vi "HFRR ADV v06.vi"() -> ()   [LabVIEW 2025] (continued)
                n1256 = property on="ENTER THE NEW PASSWORD" class="Str"("Visible"=FALSE) -> ()  [unwired: 2 in, 2 out]
              }
              frame True {
                # "password"
                # "change password logic"
                n1257 = local read "ENTER CURRENT PASSWORD"() -> (w2424:string)
                n1258 = local read "dipl pwd"() -> (w2418:string)
                n1259 = String To Byte Array(string=w2424) -> (unsigned byte array=w2426:u8[])
                n1260 = String To Byte Array(string=w2418) -> (unsigned byte array=w2419:u8[])
                n1261 = Array Size(array=w2426) -> (size(s)=w2423:i32)
                n1262 = Array Size(array=w2419) -> (size(s)=w2421:i32)
                n1263 = for {
                  N: w2423 -> [_]
                  tunnel: w2426 -> [w2450]
                  tunnel: [w2448] -> w2427 mode=indexing
                  tunnel: w2423 -> [w2442]
                  i -> [w2443]
                  n1264 = Decrement(x=w2442) -> (x-1=w2440:i32)
                  n1265 = Equal?(x=w2443, y=w2440) -> (x = y?=w2441:bool)
                  n1266 = Index Array(array=w2450, index=w2443) -> (element=w2444:u8)
                  n1267 = Number To Decimal String(number=w2444) -> (decimal integer string=w2449:string)  [unwired: 1 in]
                  n1268 = Select(t="", s=w2441, f="\r") -> (s? t:f=w2446:string)
                  n1269 = Concatenate Strings(w2449, w2446) -> (w2448:string)
                }
                n1270 = for {
                  N: w2421 -> [_]
                  tunnel: w2419 -> [w2438]
                  tunnel: [w2436] -> w2420 mode=indexing
                  tunnel: w2421 -> [w2433]
                  i -> [w2434]
                  n1271 = Decrement(x=w2433) -> (x-1=w2432:i32)
                  n1272 = Equal?(x=w2434, y=w2432) -> (x = y?=w2431:bool)
                  n1273 = Index Array(array=w2438, index=w2434) -> (element=w2437:u8)
                  n1274 = Number To Decimal String(number=w2437) -> (decimal integer string=w2435:string)  [unwired: 1 in]
                  n1275 = Select(t="", s=w2431, f="\r") -> (s? t:f=w2428:string)
                  n1276 = Concatenate Strings(w2435, w2428) -> (w2436:string)
                }
                n1277 = local read "string"() -> (w2425:string)
                n1278 = Concatenate Strings(w2420) -> (w2414:string)
                n1279 = Concatenate Strings(w2425) -> (w2422:string)
                n1280 = Concatenate Strings(w2427) -> (w2415:string)
                n1281 = Equal?(x=w2415, y=w2422) -> (x = y?=w2417:bool)
                n1282 = Equal?(x=w2415, y=w2414) -> (x = y?=w2413:bool)
                n1283 = Or(x=w2417, y=w2413) -> (x .or. y?=w2416:bool)
                n1284 = case shown="True" w2416 {
                  frame False {
                  }
                  frame True {
                    n1285 = property on="ENTER THE NEW PASSWORD" class="Str"("Visible"=TRUE) -> ()  [unwired: 2 in, 2 out]
                  }
                }
              }
            }
          }
          frame #2 {
            n1286 = String To Byte Array(string="ENTER THE NEW PASSWORD") -> (unsigned byte array=w2453:u8[])
            n1287 = Search 1D Array(1D array=w2453, element=u8 10) -> (index of element=w2457:i32)  [unwired: 1 in]
            n1288 = Index Array(array=w2453, index=w2457) -> (element=w2455:u8)
            n1289 = Equal?(x=w2455, y=10) -> (x = y?=w2452:bool)
            n1290 = case shown="False" w2452 {
              frame False {
              }
              frame True {
                n1291 = local write "EDIT"(FALSE) -> ()
                n1292 = local write "SrvM CP"(FALSE) -> ()
                n1293 = local read "ENTER THE NEW PASSWORD"() -> (w2460:string)
                n1294 = String To Byte Array(string=w2460) -> (unsigned byte array=w2465:u8[])
                n1295 = Array Size(array=w2465) -> (size(s)=w2462:i32)
                n1296 = for {
                  N: w2462 -> [_]
                  tunnel: w2465 -> [w2478]
                  tunnel: [w2475] -> w2467 mode=indexing
                  tunnel: w2462 -> [w2470]
                  i -> [w2468]
                  n1297 = Decrement(x=w2470) -> (x-1=w2471:i32)
                  n1298 = Equal?(x=w2468, y=w2471) -> (x = y?=w2472:bool)
                  n1299 = Index Array(array=w2478, index=w2468) -> (element=w2477:u8)
                  n1300 = Number To Decimal String(number=w2477) -> (decimal integer string=w2476:string)  [unwired: 1 in]
                  n1301 = Select(t="", s=w2472, f="\r") -> (s? t:f=w2469:string)
                  n1302 = Concatenate Strings(w2476, w2469) -> (w2475:string)
                }
                n1303 = local read "file path"() -> (w2459:path)
                n1304 = Concatenate Strings(w2467) -> (w2461:string)
                n1305 = Delete(path (use dialog)=w2459) -> (deleted path=w2463:path)  [unwired: 4 in, 2 out]
                n1306 = call <vilib>:"Write Characters To File.vi"("append to file? (new file:F)"=FALSE, "character string"=w2461, "file path (dialog if empty)"=w2463) -> ()  [unwired: 2 in, 1 out]
              }
            }
          }
          frame #3 {
            n1307 = case shown="True" "SrvM CP" {
              frame False {
                w2481 = ""
                n1308 = local write "ENTER CURRENT PASSWORD"(w2481) -> ()
                n1309 = local write "ENTER THE NEW PASSWORD"(w2481) -> ()
                n1310 = property on="ENTER CURRENT PASSWORD" class="Str"("Visible"=FALSE) -> ()  [unwired: 2 in, 2 out]
              }
              frame True {
                n1311 = property on="ENTER THE NEW PASSWORD" class="Str"() -> ("Visible"=w2482:bool)  [unwired: 2 in, 2 out]
                n1312 = Not(x=w2482) -> (.not. x?=w2483:bool)
                n1313 = property on="ENTER CURRENT PASSWORD" class="Str"("Visible"=w2483) -> ()  [unwired: 2 in, 2 out]
              }
            }
          }
          frame #4 {
            n1314 = String To Byte Array(string="Password") -> (unsigned byte array=w2490:u8[])
            n1315 = Search 1D Array(1D array=w2490, element=u8 10) -> (index of element=w2488:i32)  [unwired: 1 in]
            n1316 = Index Array(array=w2490, index=w2488) -> (element=w2489:u8)
            n1317 = Equal?(x=w2489, y=10) -> (x = y?=w2485:bool)
            n1318 = case shown="True" w2485 {
              frame False {
              }
              frame True {
                # "password"
                # "password"
                n1319 = local read "Password"() -> (w2503:string)
                n1320 = String To Byte Array(string=w2503) -> (unsigned byte array=w2506:u8[])
                n1321 = String To Byte Array(string="@143$\n") -> (unsigned byte array=w2492:u8[])
                n1322 = Array Size(array=w2506) -> (size(s)=w2501:i32)
                n1323 = Array Size(array=w2492) -> (size(s)=w2497:i32)
                n1324 = for {
                  N: w2501 -> [_]
                  tunnel: w2506 -> [w2523]
                  tunnel: [w2521] -> w2507 mode=indexing
                  tunnel: w2501 -> [w2518]
                  i -> [w2519]
                  n1325 = Decrement(x=w2518) -> (x-1=w2517:i32)
                  n1326 = Index Array(array=w2523, index=w2519) -> (element=w2522:u8)
                  n1327 = Equal?(x=w2519, y=w2517) -> (x = y?=w2516:bool)
                  n1328 = Number To Decimal String(number=w2522) -> (decimal integer string=w2520:string)  [unwired: 1 in]
                  n1329 = Select(t="", s=w2516, f="\r") -> (s? t:f=w2513:string)
                  n1330 = Concatenate Strings(w2520, w2513) -> (w2521:string)
                }
                n1331 = for {
                  N: w2497 -> [_]
                  tunnel: w2492 -> [w2534]
                  tunnel: [w2532] -> w2495 mode=indexing
                  tunnel: w2497 -> [w2529]
                  i -> [w2530]
                  n1332 = Decrement(x=w2529) -> (x-1=w2528:i32)
                  n1333 = Index Array(array=w2534, index=w2530) -> (element=w2533:u8)
                  n1334 = Equal?(x=w2530, y=w2528) -> (x = y?=w2527:bool)
                  n1335 = Number To Decimal String(number=w2533) -> (decimal integer string=w2531:string)  [unwired: 1 in]
                  n1336 = Select(t="", s=w2527, f="\r") -> (s? t:f=w2524:string)
                  n1337 = Concatenate Strings(w2531, w2524) -> (w2532:string)
                }
                n1338 = local read "file path"() -> (w2491:path)
                n1339 = call <vilib>:"Read Characters From File.vi"("file path (dialog if empty)"=w2491) -> ("character string"=w2505:string)  [unwired: 5 in, 3 out]
                "string" <- w2505
                n1340 = flat-sequence {
                  tunnel: [w2508] -> w2502
                  frame #0 {
                    w2508 = ""
                    n1341 = local write "Password"(w2508) -> ()
                  }
                }
                n1342 = Concatenate Strings(w2495) -> (w2496:string)
                n1343 = Concatenate Strings(w2505) -> (w2504:string)
                n1344 = Concatenate Strings(w2507) -> (w2499:string)
                n1345 = Equal?(x=w2499, y=w2504) -> (x = y?=w2494:bool)
                n1346 = Equal?(x=w2499, y=w2496) -> (x = y?=w2500:bool)
                n1347 = Or(x=w2494, y=w2500) -> (x .or. y?=w2493:bool)
                "x = y?" <- w2493
                n1348 = case shown="False" w2493 {
                  selector: w2493 -> [w2510 _]
                  tunnel: w2502 -> [_ _]
                  frame False {
                    n1349 = And(x=w2510, y=TRUE ("Visible")) -> (x .and. y?=w2511:bool)
                    n1350 = property on="message" class="Str"("Visible"=w2511) -> ()  [unwired: 2 in, 2 out]
                  }
                  frame True {
                    n1351 = property on="message" class="Str"("Visible"=FALSE) -> ()  [unwired: 2 in, 2 out]
                  }
                }
              }
            }
          }
        }
        n1352 = local read "x = y?"() -> (w2350:bool)
        n1353 = local read "HUMIDITY: 2"() -> (w2352:dbl)
        n1354 = local read "HUMIDITY:"() -> (w2351:dbl)
        n1355 = property on="Port 2 Error" class="Clust (strict)"("Visible"="EDIT") -> ()  [unwired: 2 in, 2 out]
        n1356 = property on="Port 1 Error" class="Clust (strict)"("Visible"="EDIT") -> ()  [unwired: 2 in, 2 out]
        n1357 = case shown="True" "SrvM CP 2" {
          frame False {
          }
          frame True {
            n1358 = local write "SrvM CP 2"(FALSE ("SrvM CP 2")) -> ()
            n1359 = local read "HUMIDITY: 2"() -> (w2391:dbl)
            n1360 = local read "TEMP INTERCEPT: 2"() -> (w2390:dbl)
            n1361 = local read "DISPLACEMENT : 4"() -> (w2394:dbl)
            n1362 = local read "TEMPERATURE : 2"() -> (w2393:dbl)
            n1363 = local read "STROKE GAIN : 2"() -> (w2395:dbl)
            n1364 = local read "FRIC. FORCE : 2"() -> (w2396:dbl)
            n1365 = local read "AIR TEMP INTERCEPT: 2"() -> (w2389:dbl)
            n1366 = local read "AIR TEMPERATURE : 2"() -> (w2392:dbl)
            n1367 = local write "HUMIDITY:"(w2391) -> ()
            n1368 = local write "AIR TEMP INTERCEPT:"(w2390) -> ()
            n1369 = local write "TEMPERATURE :"(w2393) -> ()
            n1370 = local write "FRIC. FORCE :"(w2396) -> ()
            n1371 = local write "STROKE GAIN :"(w2395) -> ()
            n1372 = local write "DISPLACEMENT :"(w2394) -> ()
            n1373 = local write "AIR TEMPERATURE :"(w2392) -> ()
            n1374 = local write "TEMP INTERCEPT:"(w2389) -> ()
          }
        }
        n1375 = case shown="True" "SAVE" {
          frame False {
          }
          frame True {
            n1376 = stacked-sequence {
              seq-local: [w2551 _ _] -> [_ w2715 _]
              frame #0 {
                (unwired) i16 5 ("precision (6)")
                # "[CH1]    - FF\n[CH2]   - TEMPERATURE\n[CH3]    - Humidity\n[CH4]    - AIR TEMP\n[CH5]\\- Visa Uno\n[CH6] \\- Visa Due\n[CH7]  \\- file path\n[CH8]   - Displacement Gain\n[CHA]   - Stroke Gain\n[CHB]   - Stroke PID Gain\n[CHC]   -Language Selection\n[CHD]   -Power +\n[CHE]   -Power_\n[CHF]   -Heater\n[CHG]   -Humidity Wet\n[CHH]   -Humidity Dry\n[CHI]   -Integral Time"
                n1377 = local read "Stroke PID Gains"() -> (w2602:T8)
                n1378 = Unbundle By Name(w2602) -> ("Proportional Gain (Kc)"=w2601:dbl, "Integral Time (Ti, min)"=w2543:dbl)
                n1379 = Number To Fractional String(number=w2543, width (-)=i16 10 ("precision (6)"), precision (6)=i16 5) -> (F-format string=w2547:string)  [unwired: 1 in]
                n1380 = local read "Language Selection"() -> (w2599:enum16{"English", "Russian"})
                n1381 = local read "CH-HUMIDITY WET"() -> (w2557:u16)
                n1382 = local read "CH-HUMIDITY DRY"() -> (w2554:u16)
                n1383 = local read "STROKE GAIN :"() -> (w2535:dbl)
                n1384 = local read "CH-POWER +"() -> (w2566:u16)
                n1385 = local read "CH-POWER -"() -> (w2563:u16)
                n1386 = local read "CH-HEATER"() -> (w2560:u16)
                n1387 = local read "AIR TEMPERATURE :"() -> (w2538:dbl)
                n1388 = Concatenate Strings("[CHI]" ("string"), w2547, "-Integral Time " ("string"), "\r") -> (w2544:string)
                n1389 = local read "DISPLACEMENT :"() -> (w2536:dbl)
                n1390 = local read "TEMPERATURE :"() -> (w2539:dbl)
                n1391 = local read "FRIC. FORCE :"() -> (w2540:dbl)
                n1392 = local read "HUMIDITY:"() -> (w2537:dbl)
                n1393 = Path To String(path="File Path") -> (string=w2624:string)
                n1394 = Number To Fractional String(number=w2535, width (-)=i16 10 ("precision (6)"), precision (6)=i16 5) -> (F-format string=w2615:string)  [unwired: 1 in]
                n1395 = Number To Fractional String(number=w2601, width (-)=i16 10 ("precision (6)"), precision (6)=i16 5) -> (F-format string=w2603:string)  [unwired: 1 in]
                n1396 = Number To Fractional String(number=w2599, width (-)=i16 10 ("precision (6)"), precision (6)=i16 5) -> (F-format string=w2595:string)  [unwired: 1 in]
                n1397 = Number To Fractional String(number=w2566, width (-)=i16 10 ("precision (6)"), precision (6)=i16 5) -> (F-format string=w2589:string)  [unwired: 1 in]
                n1398 = Number To Fractional String(number=w2563, width (-)=i16 10 ("precision (6)"), precision (6)=i16 5) -> (F-format string=w2586:string)  [unwired: 1 in]
                n1399 = Number To Fractional String(number=w2560, width (-)=i16 10 ("precision (6)"), precision (6)=i16 5) -> (F-format string=w2581:string)  [unwired: 1 in]
                n1400 = Number To Fractional String(number=w2557, width (-)=i16 10 ("precision (6)"), precision (6)=i16 5) -> (F-format string=w2578:string)  [unwired: 1 in]
                n1401 = Number To Fractional String(number=w2554, width (-)=i16 10 ("precision (6)"), precision (6)=i16 5) -> (F-format string=w2573:string)  [unwired: 1 in]
                n1402 = local read "Com Port 1"() -> (w2542:refnum<visa-resource-name>)
                n1403 = local read "Com Port 2"() -> (w2541:refnum<visa-resource-name>)
                n1404 = Concatenate Strings(w2624, "\\" ("string")) -> (w2623:string)
                n1405 = Number To Fractional String(number=w2540, width (-)=i16 10 ("precision (6)"), precision (6)=i16 5) -> (F-format string=w2656:string)  [unwired: 1 in]
                n1406 = Number To Fractional String(number=w2539, width (-)=i16 10 ("precision (6)"), precision (6)=i16 5) -> (F-format string=w2655:string)  [unwired: 1 in]
                n1407 = Number To Fractional String(number=w2537, width (-)=i16 10 ("precision (6)"), precision (6)=i16 5) -> (F-format string=w2649:string)  [unwired: 1 in]
                n1408 = Number To Fractional String(number=w2538, width (-)=i16 10 ("precision (6)"), precision (6)=i16 5) -> (F-format string=w2643:string)  [unwired: 1 in]
                n1409 = Number To Fractional String(number=w2536, width (-)=i16 10 ("precision (6)"), precision (6)=i16 5) -> (F-format string=w2616:string)  [unwired: 1 in]
                n1410 = Concatenate Strings("[CHA]" ("string"), w2615, "- Stroke Gain" ("string"), "\r") -> (w2609:string)
                n1411 = Concatenate Strings("[CHB]" ("string"), w2603, "- Stroke PID Gain" ("string"), "\r") -> (w2600:string)
                n1412 = Concatenate Strings("[CHC]" ("string"), w2595, "-Language Selection" ("string"), "\r") -> (w2592:string)
                n1413 = Concatenate Strings("[CHD]" ("string"), w2589, "-Power +" ("string"), "\r") -> (w2571:string)
                n1414 = Concatenate Strings("[CHG]" ("string"), w2578, "-Humidity Wet" ("string"), "\r") -> (w2568:string)
                n1415 = Concatenate Strings("[CHH]" ("string"), w2573, "-Humidity Dry" ("string"), "\r") -> (w2567:string)
                n1416 = Concatenate Strings("[CH1]" ("string"), w2656, " - FF" ("string"), "\r") -> (w2654:string)
                n1417 = Concatenate Strings("[CH2]" ("string"), w2655, " - TEMPERATURE" ("string"), "\r") -> (w2653:string)
                n1418 = Concatenate Strings("[CH3]" ("string"), w2649, " - Humidity" ("string"), "\r") -> (w2646:string)
                n1419 = Concatenate Strings("[CH4]" ("string"), w2643, " - AIR TEMP" ("string"), "\r") -> (w2639:string)
                n1420 = Concatenate Strings("[CH5]" ("string"), w2542, "- Visa Uno" ("string"), "\r") -> (w2632:string)
                n1421 = Concatenate Strings("[CH6]" ("string"), w2541, "- Visa Due" ("string"), "\r") -> (w2627:string)
                n1422 = Concatenate Strings("[CH7]" ("string"), w2623, "- file path" ("string"), "\r") -> (w2626:string)
                n1423 = Concatenate Strings("[CH8]" ("string"), w2616, "- Displacement Gain" ("string"), "\r") -> (w2619:string)
                n1424 = Concatenate Strings("[CHE]" ("string"), w2586, "-Power_" ("string"), "\r") -> (w2570:string)
                n1425 = Concatenate Strings("[CHF]" ("string"), w2581, "-Heater" ("string"), "\r") -> (w2569:string)
                n1426 = Concatenate Strings(w2654, w2653, w2646, w2639, w2632, w2627, w2626, w2619, w2609, w2600, w2592, w2571, w2570, w2569, w2568, w2567, w2544) -> (w2551:string)
                "gain" <- w2551
              }
              frame #1 {
                n1427 = local read "Camera Port :"() -> (w2668:string)
                n1428 = local read "TEMP INTERCEPT:"() -> (w2677:dbl)
                n1429 = local read "Humidity :"() -> (w2676:refnum<visa-resource-name>)
                n1430 = local read "AIR TEMP INTERCEPT:"() -> (w2678:dbl)
                n1431 = local read "LvdtOff"() -> (w2680:dbl)
                n1432 = Number To Fractional String(number=w2677, width (-)=i16 10 ("precision (6)"), precision (6)=i16 5) -> (F-format string=w2703:string)  [unwired: 1 in]
                n1433 = local read "Com Port 3"() -> (w2687:refnum<visa-resource-name>)
                n1434 = Concatenate Strings("[CH8]" ("string"), w2668, "- Visa Camera" ("string"), "\r") -> (w2667:string)
                n1435 = Concatenate Strings("[CH7]" ("string"), w2676, "- Visa Humidity" ("string"), "\r") -> (w2672:string)
                n1436 = Number To Fractional String(number=w2678, width (-)=i16 10 ("precision (6)"), precision (6)=i16 5) -> (F-format string=w2710:string)  [unwired: 1 in]
                n1437 = Number To Fractional String(number=w2680, width (-)=i16 10 ("precision (6)"), precision (6)=i16 5) -> (F-format string=w2684:string)  [unwired: 1 in]
                n1438 = Concatenate Strings("[CHK]" ("string"), w2703, "-TEMP INTERCEPT" ("string"), "\r") -> (w2699:string)
                n1439 = Concatenate Strings("[SNO]" ("string"), "S.NO", "-" ("string"), "\r") -> (w2695:string)
                n1440 = Concatenate Strings("[CHI]" ("string"), w2684, "-LVDT Position Offset" ("string"), "\r") -> (w2679:string)
                n1441 = Concatenate Strings("[CHJ]" ("string"), w2710, "-AIR TEMP INTERCEPT" ("string"), "\r") -> (w2700:string)
                n1442 = Concatenate Strings("[CHL]" ("string"), w2687, "- Visa humid" ("string"), "\r") -> (w2690:string)
                n1443 = String To Path(string="C:\\LAB-IQ\\calibrate WO 2464.dcf") -> (path=w2688:path)
                n1444 = Concatenate Strings(w2715, w2700, w2699, w2695, w2690, w2679, w2672, w2667) -> (w2714:string)
                n1445 = call <vilib>:"Write Characters To File.vi"("append to file? (new file:F)"=FALSE, "character string"=w2714, "file path (dialog if empty)"=w2688) -> ()  [unwired: 2 in, 1 out]
              }
              frame #2 {
                n1446 = local write "Lan flag"(0.0 ("Lan flag")) -> ()
                n1447 = local write "conststatus"(0.0 ("rpm value : 2")) -> ()
                n1448 = local write "SAVE"(FALSE ("OK Button 14")) -> ()
                n1449 = local write "Re-Initialise"(TRUE ("Re-Initialise")) -> ()
              }
            }
          }
        }
        n1450 = And(x="EDIT", y=w2350) -> (x .and. y?=w2348:bool)
        n1451 = local read "DISPLACEMENT : 4"() -> (w2361:dbl)
        n1452 = local read "TEMPERATURE : 2"() -> (w2359:dbl)
        n1453 = local read "STROKE GAIN : 2"() -> (w2365:dbl)
        n1454 = local read "DISPLACEMENT :"() -> (w2360:dbl)
        n1455 = local read "FRIC. FORCE : 2"() -> (w2368:dbl)
        n1456 = local read "TEMPERATURE :"() -> (w2357:dbl)
        n1457 = local read "STROKE GAIN :"() -> (w2364:dbl)
        n1458 = local read "FRIC. FORCE :"() -> (w2367:dbl)
        n1459 = case shown="False" w2348 {
          tunnel: [u8 2 ("Disabled") u8 0 ("Disabled")] -> w2347
          tunnel: [w2720 TRUE ("Visible")] -> w2346
          frame False {
            w2720 = FALSE ("Visible")
            n1460 = local write "EDIT 2"(w2720) -> ()
          }
          frame True {
          }
        }
        n1461 = Subtract(x=w2352, y=w2351) -> (x-y=w2353:dbl)
        n1462 = local read "AIR TEMPERATURE : 2"() -> (w2356:dbl)
        n1463 = local read "AIR TEMPERATURE :"() -> (w2355:dbl)
        n1464 = Divide(x=w2353, y=w2351) -> (x/y=w2375:dbl)
        n1465 = Subtract(x=w2368, y=w2367) -> (x-y=w2366:dbl)
        n1466 = Subtract(x=w2359, y=w2357) -> (x-y=w2358:dbl)
        n1467 = Subtract(x=w2365, y=w2364) -> (x-y=w2363:dbl)
        n1468 = Subtract(x=w2361, y=w2360) -> (x-y=w2362:dbl)
        n1469 = Subtract(x=w2356, y=w2355) -> (x-y=w2354:dbl)
        n1470 = Divide(x=w2366, y=w2367) -> (x/y=w2386:dbl)
        n1471 = Divide(x=w2358, y=w2357) -> (x/y=w2379:dbl)
        n1472 = Divide(x=w2363, y=w2364) -> (x/y=w2383:dbl)
        n1473 = Divide(x=w2362, y=w2360) -> (x/y=w2382:dbl)
        n1474 = Multiply(x=w2375, y=100.0) -> (x*y=→"HUMIDITY  Calibration Error":dbl)
        n1475 = Divide(x=w2354, y=w2355) -> (x/y=w2378:dbl)
        n1476 = Multiply(x=w2386, y=100.0) -> (x*y=→"FRIC. FORCE Calibration Error":dbl)
        n1477 = Multiply(x=w2379, y=100.0) -> (x*y=→"TEMPERATURE  Calibration Error":dbl)
        n1478 = Multiply(x=w2383, y=100.0) -> (x*y=→"STROKE Calibration Error":dbl)
        n1479 = Multiply(x=w2382, y=100.0) -> (x*y=→"DISPLACEMENT  Calibration Error":dbl)
        n1480 = property on="EDIT 2" class="Bool (strict)"("Visible"=w2346) -> ()  [unwired: 2 in, 2 out]
        n1481 = property on="SAVE" class="Bool (strict)"("Visible"=w2346) -> ()  [unwired: 2 in, 2 out]
        n1482 = property on="SrvM CP" class="Bool (strict)"("Disabled"=w2347) -> ()  [unwired: 2 in, 2 out]
        n1483 = property on="visa due" class="CmbBox"("Disabled"=w2347) -> ()  [unwired: 2 in, 2 out]
        n1484 = property on="LvdtOff" class="DigNum (strict)"("Disabled"=w2347) -> ()  [unwired: 2 in, 2 out]
        n1485 = property on="File Path" class="Path"("Disabled"=w2347) -> ()  [unwired: 2 in, 2 out]
        n1486 = Multiply(x=w2378, y=100.0) -> (x*y=→"AIR TEMPERATURE  Calibration Error":dbl)
        n1487 = property on="Tab Control" class="TabCtl (strict)"("Visible"=w2346) -> ()  [unwired: 2 in, 2 out]
        n1488 = property on="Language Selection" class="Enum (strict)"("Visible"=w2346) -> ()  [unwired: 2 in, 2 out]
        n1489 = property on="Tab Control 7" class="TabCtl (strict)"("Disabled"=w2347) -> ()  [unwired: 2 in, 2 out]
        n1490 = property on="AIR TEMP INTERCEPT:" class="DigNum (strict)"("Disabled"=w2347) -> ()  [unwired: 2 in, 2 out]
        n1491 = property on="CH-POWER -" class="DigNum (strict)"("Disabled"=w2347) -> ()  [unwired: 2 in, 2 out]
        n1492 = property on="CH-POWER +" class="DigNum (strict)"("Disabled"=w2347) -> ()  [unwired: 2 in, 2 out]
        n1493 = property on="AIR TEMPERATURE :" class="DigNum (strict)"("Disabled"=w2347) -> ()  [unwired: 2 in, 2 out]
        n1494 = property on="STROKE GAIN :" class="DigNum (strict)"("Disabled"=w2347) -> ()  [unwired: 2 in, 2 out]
        n1495 = property on="SPEED OUT:" class="DigNum (strict)"("Disabled"=w2347) -> ()  [unwired: 2 in, 2 out]
        n1496 = property on="CH-HUMIDITY DRY" class="DigNum (strict)"("Disabled"=w2347) -> ()  [unwired: 2 in, 2 out]
        n1497 = property on="HUMIDITY:" class="DigNum (strict)"("Disabled"=w2347) -> ()  [unwired: 2 in, 2 out]
        n1498 = property on="CH-HUMIDITY WET" class="DigNum (strict)"("Disabled"=w2347) -> ()  [unwired: 2 in, 2 out]
        n1499 = property on="Stroke PID Gains" class="Clust (strict)"("Disabled"=w2347) -> ()  [unwired: 2 in, 2 out]
        n1500 = property on="TEMPERATURE :" class="DigNum (strict)"("Disabled"=w2347) -> ()  [unwired: 2 in, 2 out]
        n1501 = property on="DISPLACEMENT :" class="DigNum (strict)"("Disabled"=w2347) -> ()  [unwired: 2 in, 2 out]
        n1502 = property on="CH-HEATER" class="DigNum (strict)"("Disabled"=w2347) -> ()  [unwired: 2 in, 2 out]
        n1503 = property on="TEMP INTERCEPT:" class="DigNum (strict)"("Disabled"=w2347) -> ()  [unwired: 2 in, 2 out]
        n1504 = property on="FRIC. FORCE :" class="DigNum (strict)"("Disabled"=w2347) -> ()  [unwired: 2 in, 2 out]
      }
    }
    n1505 = local read "Re-Initialise"() -> (w1729:bool)
    n1506 = local read "Main Tab"() -> (w1725:T2)
    n1507 = local read "service 3"() -> (w1726:bool)
    n1508 = local read "OPEN 6"() -> (w1728:bool)
    n1509 = local read "EDIT 2"() -> (w1731:bool)
    n1510 = local read "RUN"() -> (w1743:bool)
    n1511 = local read "RUN"() -> (w1741:bool)
    n1512 = disable-structure shown="Disabled" {
      disable-tunnel: [w1758 _] -> w1723
      disable-tunnel: [w1757 _] -> w1721
      frame Disabled {
        n1513 = local read "Temperature before test"() -> (w1751:dbl)
        n1514 = local read "Temperature after test"() -> (w1764:dbl)
        n1515 = case shown="True" "Save Results" {
          frame False {
          }
          frame True {
            w1780 = "\r"
            n1516 = local write "Save Results"(FALSE ("OK Button 5")) -> ()
            n1517 = local read "Temperature before test"() -> (w1818:dbl)
            n1518 = local read "Temperature after test"() -> (w1820:dbl)
            n1519 = local read "Humidity before test"() -> (w1817:dbl)
            n1520 = local read "Humidity after test"() -> (w1819:dbl)
            n1521 = local read "WS1.4"() -> (w1824:dbl)
            n1522 = local read "AVP"() -> (w1822:dbl)
            n1523 = Number To Fractional String(number=w1824, width (-)=i16 6, precision (6)=i16 1) -> (F-format string=w1784:string)  [unwired: 1 in]
            n1524 = local read "MWSD"() -> (w1821:dbl)
            n1525 = local read "String"() -> (w1813:string)
            n1526 = local read "FILE"() -> (w1816:string)
            n1527 = local read "HCF"() -> (w1823:dbl)
            n1528 = Number To Fractional String(number=w1817, width (-)=i16 6, precision (6)=i16 1) -> (F-format string=w1809:string)  [unwired: 1 in]
            n1529 = Number To Fractional String(number=w1818, width (-)=i16 6, precision (6)=i16 1) -> (F-format string=w1806:string)  [unwired: 1 in]
            n1530 = Number To Fractional String(number=w1819, width (-)=i16 6, precision (6)=i16 1) -> (F-format string=w1802:string)  [unwired: 1 in]
            n1531 = Number To Fractional String(number=w1820, width (-)=i16 6, precision (6)=i16 1) -> (F-format string=w1798:string)  [unwired: 1 in]
            n1532 = Number To Fractional String(number=w1822, width (-)=i16 6, precision (6)=i16 3) -> (F-format string=w1791:string)  [unwired: 1 in]
            n1533 = Concatenate Strings(w1813, w1816) -> (w1835:string)
            n1534 = Number To Fractional String(number=w1821, width (-)=i16 6, precision (6)=i16 1) -> (F-format string=w1795:string)  [unwired: 1 in]
            n1535 = Number To Fractional String(number=w1823, width (-)=i16 6, precision (6)=i16 2) -> (F-format string=w1789:string)  [unwired: 1 in]
            n1536 = Concatenate Strings("(" ("string"), w1784, ")Microns" ("string")) -> (w1783:string)
            n1537 = local read "REMARKS"() -> (w1815:string)
            "REMARKS 2" <- w1815
            n1538 = Concatenate Strings("(" ("string"), w1809, " ) % RH," ("string")) -> (w1810:string)
            n1539 = Concatenate Strings(w1789, ")" ("string")) -> (w1787:string)
            n1540 = Concatenate Strings("(" ("string"), w1806, ")  Deg C ," ("string")) -> (w1805:string)
            n1541 = Concatenate Strings("(" ("string"), w1802, " ) % RH," ("string")) -> (w1801:string)
            n1542 = Concatenate Strings("(" ("string"), w1798, ")  Deg C ," ("string")) -> (w1797:string)
            n1543 = Concatenate Strings("(" ("string"), w1795, ")  Microns," ("string")) -> (w1794:string)
            n1544 = Concatenate Strings("(" ("string"), w1791, ")  kPa," ("string")) -> (w1781:string)
            n1545 = Concatenate Strings(w1835, ".dwm" ("Substring")) -> (w1833:string)
            n1546 = String To Path(string=w1833) -> (path=w1832:path)
            n1547 = Concatenate Strings(w1815, w1780, " Humidity before test= " ("Substring"), w1810, w1780, " Temperature before test = " ("Substring"), w1805, w1780, " Humidity after test= " ("Substring"), w1801, w1780, "Temperature after test = " ("Substring"), w1797, w1780, "MSD = " ("Substring"), w1794, w1780, "  AVP = " ("Substring"), w1781, w1780, "  HCF                     =( " ("Substring"), w1787, w1780, " WS1.4                  = " ("Substring"), w1783, w1780) -> (w1779:string)
            "data" <- w1779
            n1548 = call <vilib>:"Write Characters To File.vi"("append to file? (new file:F)"=FALSE, "character string"=w1779, "file path (dialog if empty)"=w1832) -> ()  [unwired: 2 in, 1 out]
            n1549 = Match Pattern(string=w1779, regular expression="!") -> (after substring=→"export":string)  [unwired: 1 in, 3 out]
          }
        }
        n1550 = Add(x=231.864, y=w1751) -> (x+y=w1748:dbl)
        n1551 = Add(x=231.864, y=w1764) -> (x+y=w1761:dbl)
        n1552 = Divide(x=1705.984, y=w1748) -> (x/y=w1749:dbl)
        n1553 = Divide(x=1705.984, y=w1761) -> (x/y=w1762:dbl)
        n1554 = local read "Humidity before test"() -> (w1753:dbl)
        n1555 = local read "Humidity after test"() -> (w1766:dbl)
        n1556 = Subtract(x=8.017352 ("y"), y=w1749) -> (x-y=w1775:dbl)
        n1557 = Subtract(x=8.017352 ("y"), y=w1762) -> (x-y=w1769:dbl)
        n1558 = expression code="10**y"(w1775) -> (w1755:dbl)
        n1559 = expression code="10**y"(w1769) -> (w1768:dbl)
        n1560 = Multiply(x=w1753, y=w1755) -> (x*y=w1754:dbl)
        n1561 = Multiply(x=w1766, y=w1768) -> (x*y=w1767:dbl)
        n1562 = Divide(x=w1754, y=750.0) -> (x/y=w1770:dbl)
        n1563 = Divide(x=w1767, y=750.0) -> (x/y=w1771:dbl)
        n1564 = Add(x=w1770, y=w1771) -> (x+y=w1772:dbl)
        n1565 = Divide(x=w1772, y=2.0) -> (x/y=w1774:dbl)
        n1566 = local write "AVP"(w1774) -> ()
        n1567 = Subtract(x=1.4, y=w1774) -> (x-y=w1757:dbl)
        n1568 = local read "HCF"() -> (w1758:dbl)
      }
      frame Enabled {
      }
    }
    n1569 = case shown="True" "EDIT 3" {
      frame False {
      }
      frame True {
        n1570 = local write "EDIT 3"(FALSE ("EDIT 3")) -> ()
        n1571 = local write "Main Tab"(T2."About" ("Main Tab")) -> ()
      }
    }
    n1572 = case shown="True" w1729 {
      frame False {
      }
      frame True {
        n1573 = local write "Re-Initialise"(FALSE ("Re-Initialise")) -> ()
      }
    }
    n1574 = case shown="False" w1743 {
      frame False {
        n1575 = local read "stopT"() -> (w2729:bool)
        n1576 = case shown="True" w2729 {
          frame False {
          }
          frame True {
            w2730 = FALSE
            n1577 = local write "stopT"(w2730) -> ()
            n1578 = local write "st enable"(w2730) -> ()
          }
        }
      }
      frame True {
        "stopT" <- TRUE
      }
    }
    n1579 = case shown="True" w1741 {
      frame False {
      }
      frame True {
        n1580 = local read "Main Tab"() -> (w2727:T2)
        n1581 = case shown="\"Compare Files\"" w2727 {
          frame "Acquire", Default {
          }
          frame "Compare Files" {
            n1582 = local write "Main Tab"(T2."Acquire" ("Main Tab")) -> ()
          }
          frame "About" {
          }
        }
      }
    }
    n1583 = case shown="True" w1731 {
      frame False {
        n1584 = property on="Password 2" class="Str"("Visible"=FALSE) -> ()  [unwired: 2 in, 2 out]
        n1585 = local write "Password 2"("" ("Password")) -> ()
      }
      frame True {
        n1586 = property on="Password 2" class="Str"("Visible"=TRUE) -> ()  [unwired: 2 in, 2 out]
        n1587 = Equal?(x="Password 2", y="HFRR1234") -> (x = y?=w1864:bool)
        n1588 = case shown="True" w1864 {
          tunnel: "Password 2" -> [w1867 _]
          frame False {
            n1589 = String Length(string=w1867) -> (length=w1868:i32)
            n1590 = Greater Than 0?(x=w1868) -> (x > 0?=w1866:bool)
            n1591 = case shown="False" w1866 {
              frame False {
                n1592 = property on="Password 2" class="Str"("Caption.Text"="Password (Advance Setting)") -> ()  [unwired: 2 in, 2 out]
              }
              frame True {
                n1593 = property on="Password 2" class="Str"("Caption.Text"="Incorrect Password!") -> ()  [unwired: 2 in, 2 out]
              }
            }
          }
          frame True {
            n1594 = local write "EDIT 2"(FALSE ("EDIT 2")) -> ()
            n1595 = local write "Password 2"("" ("Password")) -> ()
            n1596 = local write "Main Tab"(T2."Advance" ("Main Tab")) -> ()
          }
        }
      }
    }
    n1597 = case shown="True" "Prog Uno" {
      frame False {
      }
      frame True {
        n1598 = stacked-sequence {
          frame #0 {
            n1599 = Delete(path (use dialog)=path "C:/LAB-IQ-NXT/UNOCOMPILE.bat" ("working directory")) -> ()  [unwired: 4 in, 3 out]
          }
          frame #1 {
            n1600 = local read "Com Port 1"() -> (w2328:refnum<visa-resource-name>)
            n1601 = Concatenate Strings("cmd.exe /c \"mode " ("command line"), w2328, ":1200,n,8,1\"\n" ("command line")) -> (w2333:string)
            n1602 = Concatenate Strings(w2333, "CD\\\nCD WinDucom\navrdude -C avrdude.conf -v -patmega328p -carduino -P" ("command line"), w2328, " -b115200 -D -Uflash:w:UNO_V20.hex:i\n" ("command line"), "\r") -> (w2335:string)
            "STR" <- w2335
            n1603 = call <vilib>:"Write Characters To File.vi"("append to file? (new file:F)"=FALSE, "character string"=w2335, "file path (dialog if empty)"=path "C:/LAB-IQ-NXT/UNOCOMPILE.bat" ("working directory")) -> ()  [unwired: 2 in, 1 out]
          }
          frame #2 {
            n1604 = disable-structure shown="Disabled" {
              frame Disabled {
                w2339 = "cmd.exe  /c \"C:\\LAB-IQ-NXT\\UNOCOMPILE.bat\"" ("string")
                n1605 = local write "Prog Uno"(FALSE ("run minimized? (F)")) -> ()
                n1606 = call <vilib>:"System Exec.vi"("expected output size  (4096)"=u32 65535, "run minimized? (F)"=FALSE, "wait until completion? (T)"=TRUE ("run minimized? (F)"), "working directory"=path "C:/LAB-IQ-NXT", "standard input"=w2339, "command line"=w2339) -> ("error out"=w2338:errorcluster, "standard output"=→"String 42":string)  [unwired: 2 in, 2 out]
                "error out 3" <- w2338
                n1607 = flat-sequence {
                  tunnel: w2338 -> [_]
                  frame #0 {
                  }
                }
              }
              frame Enabled {
              }
            }
          }
        }
      }
    }
    n1608 = case shown="\"ASTM D6079\", Default" "TEST STANDARD" {
      tunnel: [2.0 ("Set Temp") 0.0 ("Set Temp") 2.0 ("Set Temp") 0.0 ("Set Temp")] -> w1732
      frame "ASTM D6079", Default {
        w2285 = 50.0 ("Hz")
        w2286 = 53.0 ("Set Rh")
        w2288 = 1.0 ("Set Strk")
        w2287 = 60.0 ("Set Temp")
        # "astm hide"
        n1609 = local write "NORMAL LOAD"(2.0 ("NORMAL LOAD")) -> ()
        n1610 = local write "Set Strk"(w2288) -> ()
        n1611 = local write "Set Hz"(w2285) -> ()
        n1612 = local write "Set Temp"(w2287) -> ()
        n1613 = local write "Set Rh"(w2286) -> ()
        n1614 = local write "test time"(75.0 ("test time")) -> ()
        n1615 = local write "Set Stroke:"(w2288) -> ()
        n1616 = local write "Set Humidity:"(w2286) -> ()
        n1617 = local write "Set Frequency:"(w2285) -> ()
        n1618 = local write "Set Temperature:"(w2287) -> ()
        "Test Standard" <- "ASTM D6079" ("Test Standard 2")
      }
      frame "ISO 12156" {
        n1619 = local write "Set Strk"(1.0 ("Set Strk")) -> ()
        n1620 = local write "NORMAL LOAD"(2.0 ("NORMAL LOAD")) -> ()
        n1621 = local write "Set Temp"(60.0 ("Set Temp")) -> ()
        n1622 = local write "test time"(75.0 ("test time")) -> ()
        n1623 = local write "Set Hz"(50.0 ("Hz")) -> ()
        n1624 = local write "Set Rh"(53.0 ("Set Rh")) -> ()
      }
      frame "CEC F-096-A-06" {
        n1625 = local write "Set Strk"(1.0 ("Set Strk")) -> ()
        n1626 = local write "NORMAL LOAD"(2.0 ("NORMAL LOAD")) -> ()
        n1627 = local write "Set Temp"(60.0 ("Set Temp")) -> ()
        n1628 = local write "test time"(75.0 ("test time")) -> ()
        n1629 = local write "Set Hz"(50.0 ("Hz")) -> ()
        n1630 = local write "Set Rh"(53.0 ("Set Rh")) -> ()
      }
      frame "Custom" {
      }
    }
    n1631 = case shown="True" "Prog Due" {
      frame False {
      }
      frame True {
        n1632 = stacked-sequence {
          frame #0 {
            n1633 = Delete(path (use dialog)=path "C:/LAB-IQ/DUECOMPILE.bat" ("working directory")) -> ()  [unwired: 4 in, 3 out]
          }
          frame #1 {
            n1634 = disable-structure shown="Disabled" {
              frame Disabled {
                n1635 = local read "visa due"() -> (w2310:string)
                n1636 = Concatenate Strings("cmd.exe /c \"mode " ("command line"), w2310, ":1200,n,8,1\"\n" ("command line")) -> (w2315:string)
                n1637 = Concatenate Strings(w2315, "CD\\\nCD WinDucom\nTIMEOUT 1\n bossac.exe -i -d --port=" ("command line"), w2310, " -U false -e -w -v -b DUE.bin -R\n" ("command line"), "\r") -> (w2317:string)
                "concatenated string 2" <- w2317
                n1638 = call <vilib>:"Write Characters To File.vi"("append to file? (new file:F)"=FALSE, "character string"=w2317, "file path (dialog if empty)"=path "C:/LAB-IQ-NXT/DUECOMPILE.bat" ("working directory")) -> ()  [unwired: 2 in, 1 out]
              }
              frame Enabled {
              }
            }
          }
          frame #2 {
            # "C:\\LAB-IQ-NXT\\DUECOMPILE.bat"
            n1639 = disable-structure shown="Disabled" {
              frame Disabled {
                w2322 = "cmd.exe  /c \"C:\\LAB-IQ-NXT\\DUECOMPILE.bat\"" ("string")
                n1640 = call <vilib>:"System Exec.vi"("expected output size  (4096)"=u32 65535, "run minimized? (F)"=FALSE, "wait until completion? (T)"=TRUE ("run minimized? (F)"), "working directory"=path "C:/LAB-IQ-NXT", "standard input"=w2322, "command line"=w2322) -> ("error out"=w2321:errorcluster, "standard output"=→"String 44":string)  [unwired: 2 in, 2 out]
                "error out 4" <- w2321
                n1641 = flat-sequence {
                  tunnel: w2321 -> [_]
                  frame #0 {
                  }
                }
              }
              frame Enabled {
              }
            }
            n1642 = local write "Prog Due"(FALSE ("Prog Due")) -> ()
          }
        }
      }
    }
    n1643 = Or(x=w1728, y=w1726) -> (x .or. y?=w1727:bool)
    n1644 = case shown="\"About\"" w1725 {
      tunnel: [T18."Acquire" ("Main Tab") T18."Compare Files" ("Main Tab") T18."About" ("Main Tab")] -> w1739
      frame "Acquire", Default {
      }
      frame "Compare Files" {
      }
      frame "About" {
      }
    }
    n1645 = Or(x=w1733, y="OPEN") -> (x .or. y?=w1734:bool)
    n1646 = case shown="True" w1734 {
      tunnel: w1733 -> [_ w1874]
      frame False {
      }
      frame True {
        n1647 = stacked-sequence {
          tunnel: w1874 -> [_ w1941 _ _]
          frame #0 {
            w1890 = "  " ("String 6")
            n1648 = local write "OPEN"(FALSE ("open")) -> ()
            n1649 = local read "string1 2"() -> (w1878:string)
            n1650 = local read "string1 3"() -> (w1877:string)
            n1651 = local read "string1 4"() -> (w1876:string)
            n1652 = property on="OPEN" class="Bool (strict)"("Visible"=FALSE) -> ()  [unwired: 2 in, 2 out]
            n1653 = local write "String 6"(w1890) -> ()
            n1654 = local write "String 7"(w1890) -> ()
            n1655 = local write "String 8"(w1890) -> ()
            n1656 = local write "String 12"(w1890) -> ()
            n1657 = local read "OK Button 16"() -> (w1875:bool)
            n1658 = String To Path(string=w1878) -> (path=w1886:path)
            n1659 = String To Path(string=w1877) -> (path=w1885:path)
            n1660 = String To Path(string=w1876) -> (path=w1884:path)
            n1661 = case shown="True" w1875 {
              tunnel: [w1891 w1892] -> w1879
              frame False {
                n1662 = local read "string1"() -> (w1891:string)
              }
              frame True {
                n1663 = local read "String Indicator 4"() -> (w1892:string)
              }
            }
            n1664 = Open/Create/Replace File "Open File"(file path (use dialog)=w1886) -> (refnum out=w1882:refnum<file>)  [unwired: 5 in, 2 out]
            n1665 = Open/Create/Replace File "Open File"(file path (use dialog)=w1885) -> (refnum out=w1881:refnum<file>)  [unwired: 5 in, 2 out]
            n1666 = Open/Create/Replace File "Open File"(file path (use dialog)=w1884) -> (refnum out=w1880:refnum<file>)  [unwired: 5 in, 2 out]
            n1667 = while {
              tunnel: w1882 -> [w1904]
              i -> [w1900]
              stop <- w1899 continue-if-true
              (unwired) TRUE ("line mode (F)")
              n1668 = Read from Text File "Read File"(file (use dialog)=w1904) -> (text=w1901:string)  [unwired: 3 in, 3 out]
              n1669 = local write "Numeric 11"(w1900) -> ()
              n1670 = String Length(string=w1901) -> (length=w1903:i32)
              n1671 = Greater?(x=w1903, y=1) -> (0:w1899:bool)
            }
            n1672 = while {
              tunnel: w1881 -> [w1910]
              i -> [w1906]
              stop <- w1905 continue-if-true
              (unwired) TRUE ("line mode (F)")
              n1673 = Read from Text File "Read File"(file (use dialog)=w1910) -> (text=w1907:string)  [unwired: 3 in, 3 out]
              n1674 = local write "Numeric 12"(w1906) -> ()
              n1675 = String Length(string=w1907) -> (length=w1909:i32)
              n1676 = Greater?(x=w1909, y=1) -> (0:w1905:bool)
            }
            n1677 = while {
              tunnel: w1880 -> [w1916]
              i -> [w1912]
              stop <- w1911 continue-if-true
              (unwired) TRUE ("line mode (F)")
              n1678 = Read from Text File "Read File"(file (use dialog)=w1916) -> (text=w1913:string)  [unwired: 3 in, 3 out]
              n1679 = local write "Numeric 13"(w1912) -> ()
              n1680 = String Length(string=w1913) -> (length=w1915:i32)
              n1681 = Greater?(x=w1915, y=1) -> (0:w1911:bool)
            }
            n1682 = String To Path(string=w1879) -> (path=w1887:path)
            n1683 = Open/Create/Replace File "Open File"(file path (use dialog)=w1887) -> (refnum out=w1883:refnum<file>)  [unwired: 5 in, 2 out]
            n1684 = while {
              tunnel: w1883 -> [w1898]
              i -> [w1894]
              stop <- w1893 continue-if-true
              (unwired) TRUE ("line mode (F)")
              n1685 = Read from Text File "Read File"(file (use dialog)=w1898) -> (text=w1895:string)  [unwired: 3 in, 3 out]
              n1686 = local write "Numeric 8"(w1894) -> ()
              n1687 = String Length(string=w1895) -> (length=w1897:i32)
              n1688 = Greater?(x=w1897, y=1) -> (0:w1893:bool)
            }
          }
          frame #1 {
            w2068 = FALSE ("ACTUAL   MERGE")
            # "Sample Temp"
            # "ECR"
            # "COF"
            # "Time\nCOF\nFF\nTemp"
            n1689 = case shown="True" w1941 {
              tunnel: [w2088 w2089] -> w1942
              frame False {
                n1690 = local read "string1"() -> (w2088:string)
              }
              frame True {
                n1691 = local read "String Indicator 4"() -> (w2089:string)
              }
            }
            n1692 = local read "string1 3"() -> (w1986:string)
            n1693 = String To Path(string=w1942) -> (path=w2073:path)
            n1694 = String To Path(string=w1986) -> (path=w2084:path)
            n1695 = local read "Numeric 12"() -> (w2070:i32)
            n1696 = local read "Numeric 8"() -> (w2072:i32)
            n1697 = local read "string1 2"() -> (w1987:string)
            n1698 = local read "string1 4"() -> (w1985:string)
            n1699 = Open/Create/Replace File "Open File"(file path (use dialog)=w2073) -> (refnum out=w2087:refnum<file>, error out=w2086:errorcluster)  [unwired: 5 in, 1 out]
            n1700 = Open/Create/Replace File "Open File"(file path (use dialog)=w2084) -> (refnum out=w2080:refnum<file>, error out=w2081:errorcluster)  [unwired: 5 in, 1 out]
            n1701 = for {
              N: w2072 -> [_]
              tunnel: w2087 -> [w2235]
              tunnel: w2086 -> [w2234]
              tunnel: [w2224] -> w1999 mode=indexing
              tunnel: [w2222] -> w2056 mode=indexing
              tunnel: [w2223] -> w2051 mode=indexing
              tunnel: w2068 -> [_]
              tunnel: [w2216] -> w2053 mode=indexing
              tunnel: [w2212] -> w2022 mode=indexing
              tunnel: [w2208] -> w1997 mode=indexing
              tunnel: [w2204] -> w1978 mode=indexing
              tunnel: [w2199] -> w1938 mode=indexing
              (unwired) TRUE ("line mode (F)")
              # "freq"
              # "Stroke"
              # "Time"
              # "CoF"
              # "Humidity"
              # "Temp"
              # "Air Temp"
              # "ECR"
              n1702 = Read from Text File "Read File"(file (use dialog)=w2235, error in=w2234) -> (text=w2200:string)  [unwired: 2 in, 3 out]
              n1703 = local write "String 6"(w2200) -> ()
              n1704 = String Subset(string=w2200, offset (0)=0, length (rest)=14 ("length (rest)")) -> (substring=w2228:string)
              n1705 = String Subset(string=w2200, offset (0)=35, length (rest)=9 ("length (rest)")) -> (substring=w2225:string)
              n1706 = String Subset(string=w2200, offset (0)=15, length (rest)=9 ("length (rest)")) -> (substring=w2231:string)
              n1707 = Fract/Exp String To Number(string=w2228) -> (number=w2224:dbl)  [unwired: 3 in, 1 out]
              n1708 = Fract/Exp String To Number(string=w2225) -> (number=w2223:dbl)  [unwired: 3 in, 1 out]
              n1709 = Fract/Exp String To Number(string=w2231) -> (number=w2222:dbl)  [unwired: 3 in, 1 out]
              n1710 = String Subset(string=w2200, offset (0)=85, length (rest)=9 ("length (rest)")) -> (substring=w2201:string)
              n1711 = String Subset(string=w2200, offset (0)=25, length (rest)=9 ("length (rest)")) -> (substring=w2207:string)
              n1712 = String Subset(string=w2200, offset (0)=55, length (rest)=9 ("length (rest)")) -> (substring=w2209:string)
              n1713 = String Subset(string=w2200, offset (0)=45, length (rest)=9 ("length (rest)")) -> (substring=w2215:string)
              n1714 = String Subset(string=w2200, offset (0)=65, length (rest)=9 ("length (rest)")) -> (substring=w2221:string)
              n1715 = Fract/Exp String To Number(string=w2207) -> (number=w2204:dbl)  [unwired: 3 in, 1 out]
              n1716 = Fract/Exp String To Number(string=w2201) -> (number=w2199:dbl)  [unwired: 3 in, 1 out]
              n1717 = Fract/Exp String To Number(string=w2209) -> (number=w2208:dbl)  [unwired: 3 in, 1 out]
              n1718 = Fract/Exp String To Number(string=w2215) -> (number=w2212:dbl)  [unwired: 3 in, 1 out]
              n1719 = Fract/Exp String To Number(string=w2221) -> (number=w2218:dbl)  [unwired: 3 in, 1 out]
              n1720 = Add(x=w2218, y=0.0) -> (x+y=w2216:dbl)
            }
            n1721 = for {
              N: w2070 -> [_]
              tunnel: w2081 -> [w2161]
              tunnel: w2080 -> [w2160]
              tunnel: [w2150] -> w2039 mode=indexing
              tunnel: [w2148] -> w2037 mode=indexing
              tunnel: [w2149] -> w2033 mode=indexing
              tunnel: w2068 -> [_]
              tunnel: [w2142] -> w2035 mode=indexing
              tunnel: [w2138] -> w2017 mode=indexing
              tunnel: [w2134] -> w1993 mode=indexing
              tunnel: [w2131] -> w1974 mode=indexing
              tunnel: [w2127] -> w1933 mode=indexing
              (unwired) 9 ("length (rest)")
              (unwired) 9 ("length (rest)")
              (unwired) TRUE ("line mode (F)")
              n1722 = Read from Text File "Read File"(file (use dialog)=w2160, error in=w2161) -> (text=w2128:string)  [unwired: 2 in, 3 out]
              n1723 = local write "String 8"(w2128) -> ()
              n1724 = String Subset(string=w2128, offset (0)=85) -> (substring=w2130:string)  [unwired: 1 in]
              n1725 = String Subset(string=w2128, offset (0)=35, length (rest)=9 ("length (rest)")) -> (substring=w2151:string)
              n1726 = String Subset(string=w2128, offset (0)=55, length (rest)=9 ("length (rest)")) -> (substring=w2136:string)
              n1727 = String Subset(string=w2128, offset (0)=25) -> (substring=w2132:string)  [unwired: 1 in]
              n1728 = String Subset(string=w2128, offset (0)=15, length (rest)=9 ("length (rest)")) -> (substring=w2157:string)
              n1729 = String Subset(string=w2128, offset (0)=0, length (rest)=14 ("length (rest)")) -> (substring=w2154:string)
              n1730 = String Subset(string=w2128, offset (0)=45, length (rest)=9 ("length (rest)")) -> (substring=w2141:string)
              n1731 = String Subset(string=w2128, offset (0)=65, length (rest)=9 ("length (rest)")) -> (substring=w2147:string)
              n1732 = Fract/Exp String To Number(string=w2130) -> (number=w2127:dbl)  [unwired: 3 in, 1 out]
              n1733 = Fract/Exp String To Number(string=w2151) -> (number=w2149:dbl)  [unwired: 3 in, 1 out]
              n1734 = Fract/Exp String To Number(string=w2136) -> (number=w2134:dbl)  [unwired: 3 in, 1 out]
              n1735 = Fract/Exp String To Number(string=w2132) -> (number=w2131:dbl)  [unwired: 3 in, 1 out]
              n1736 = Fract/Exp String To Number(string=w2157) -> (number=w2148:dbl)  [unwired: 3 in, 1 out]
              n1737 = Fract/Exp String To Number(string=w2154) -> (number=w2150:dbl)  [unwired: 3 in, 1 out]
              n1738 = Fract/Exp String To Number(string=w2141) -> (number=w2138:dbl)  [unwired: 3 in, 1 out]
              n1739 = Fract/Exp String To Number(string=w2147) -> (number=w2144:dbl)  [unwired: 3 in, 1 out]
              n1740 = Add(x=w2144, y=0.0) -> (x+y=w2142:dbl)
            }
            n1741 = String To Path(string=w1987) -> (path=w2085:path)
            n1742 = String To Path(string=w1985) -> (path=w2079:path)
            n1743 = local read "Numeric 11"() -> (w2069:i32)
            n1744 = local read "Numeric 13"() -> (w2071:i32)
            n1745 = Open/Create/Replace File "Open File"(file path (use dialog)=w2085) -> (refnum out=w2083:refnum<file>, error out=w2082:errorcluster)  [unwired: 5 in, 1 out]
            n1746 = Open/Create/Replace File "Open File"(file path (use dialog)=w2079) -> (refnum out=w2078:refnum<file>, error out=w2077:errorcluster)  [unwired: 5 in, 1 out]
            n1747 = for {
              N: w2069 -> [_]
              tunnel: w2083 -> [w2198]
              tunnel: w2082 -> [w2197]
              tunnel: [w2187] -> w2049 mode=indexing
              tunnel: [w2185] -> w2047 mode=indexing
              tunnel: [w2186] -> w2042 mode=indexing
              tunnel: w2068 -> [_]
              tunnel: [w2179] -> w2044 mode=indexing
              tunnel: [w2175] -> w2020 mode=indexing
              tunnel: [w2171] -> w1995 mode=indexing
              tunnel: [w2167] -> w1976 mode=indexing
              tunnel: [w2162] -> w1934 mode=indexing
              (unwired) TRUE ("line mode (F)")
              n1748 = Read from Text File "Read File"(file (use dialog)=w2198, error in=w2197) -> (text=w2163:string)  [unwired: 2 in, 3 out]
              n1749 = local write "String 7"(w2163) -> ()
              n1750 = String Subset(string=w2163, offset (0)=85, length (rest)=9 ("length (rest)")) -> (substring=w2166:string)
              n1751 = String Subset(string=w2163, offset (0)=35, length (rest)=9 ("length (rest)")) -> (substring=w2188:string)
              n1752 = String Subset(string=w2163, offset (0)=55, length (rest)=9 ("length (rest)")) -> (substring=w2174:string)
              n1753 = String Subset(string=w2163, offset (0)=25, length (rest)=9 ("length (rest)")) -> (substring=w2168:string)
              n1754 = String Subset(string=w2163, offset (0)=45, length (rest)=9 ("length (rest)")) -> (substring=w2176:string)
              n1755 = String Subset(string=w2163, offset (0)=0, length (rest)=14 ("length (rest)")) -> (substring=w2191:string)
              n1756 = String Subset(string=w2163, offset (0)=15, length (rest)=9 ("length (rest)")) -> (substring=w2194:string)
              n1757 = String Subset(string=w2163, offset (0)=65, length (rest)=9 ("length (rest)")) -> (substring=w2180:string)
              n1758 = Fract/Exp String To Number(string=w2166) -> (number=w2162:dbl)  [unwired: 3 in, 1 out]
              n1759 = Fract/Exp String To Number(string=w2188) -> (number=w2186:dbl)  [unwired: 3 in, 1 out]
              n1760 = Fract/Exp String To Number(string=w2174) -> (number=w2171:dbl)  [unwired: 3 in, 1 out]
              n1761 = Fract/Exp String To Number(string=w2168) -> (number=w2167:dbl)  [unwired: 3 in, 1 out]
              n1762 = Fract/Exp String To Number(string=w2176) -> (number=w2175:dbl)  [unwired: 3 in, 1 out]
              n1763 = Fract/Exp String To Number(string=w2191) -> (number=w2187:dbl)  [unwired: 3 in, 1 out]
              n1764 = Fract/Exp String To Number(string=w2194) -> (number=w2185:dbl)  [unwired: 3 in, 1 out]
